vi "TestExec.Test ID - Inc.vi"(9 "TC Level":i32, 10 "TC Cnts":i32[](array[numeric])) -> (0 "Test ID":string, 1 "TC Level Out":i32, 2 "TC Cnts Out":i32[](array[numeric]))   [LabVIEW 2016]
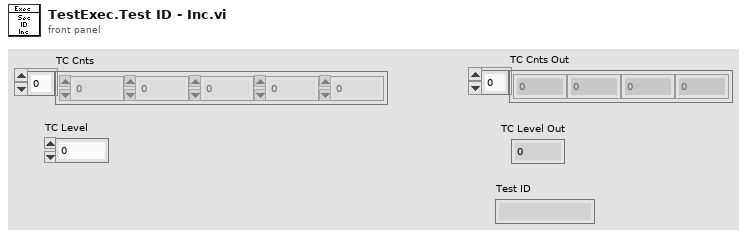
[diagram p1: front panel]
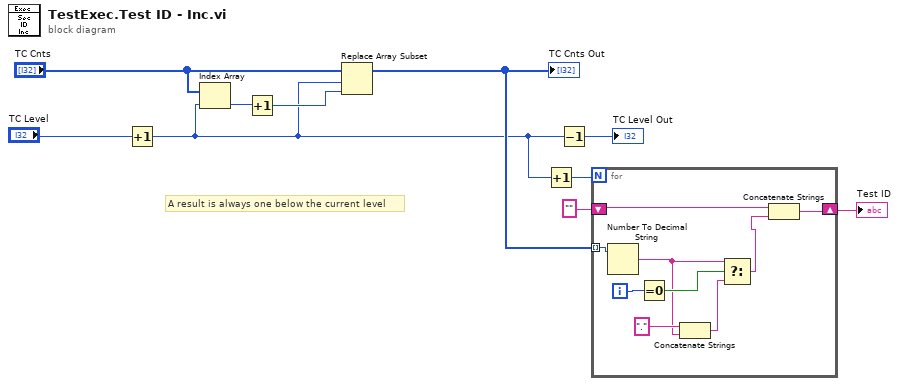
[diagram p0: block diagram]
diagram:
  # "A result is always one below the current level"
  n1 = Increment(x="TC Level") -> (x+1=w1:i32)
  n2 = Index Array(array="TC Cnts", index=w1) -> (element=w5:i32)
  n3 = Increment(x=w5) -> (x+1=w4:i32)
  n4 = Replace Array Subset(array="TC Cnts", new element=w4, index=w1) -> (w10:i32[])
  "TC Cnts Out" <- w10
  n5 = Increment(x=w1) -> (x+1=w9:i32)
  n6 = Decrement(x=w1) -> (x-1=→"TC Level Out":i32)
  n7 = for {
    N: w9 -> [_]
    tunnel: w10 -> [w18] mode=indexing
    shift-right: [w13] -> w7
    shift-left: "" -> [w12]
    i -> [w19]
    n8 = Number To Decimal String(number=w18) -> (decimal integer string=w14:string)  [unwired: 1 in]
    n9 = Equal To 0?(x=w19) -> (x = 0?=w15:bool)
    n10 = Concatenate Strings(".", w14) -> (w16:string)
    n11 = Select(t=w14, s=w15, f=w16) -> (s? t:f=w11:string)
    n12 = Concatenate Strings(w12, w11) -> (w13:string)
  }
  "Test ID" <- w7
